vi "Main.vi"() -> ()   [LabVIEW 2013]
uses:
  <vilib>/myRIO/Instrument Drivers/Onboard IO/AI/vis/Smart Open.vi
  <vilib>/myRIO/Instrument Drivers/Onboard IO/AI/vis/Read.vi
  <vilib>/myRIO/Common/Instrument Driver Framework/myRIO v1.0/UART/vis/myRIO v1.0 Close UART.vi
  <vilib>/myRIO/Instrument Drivers/Onboard IO/AI/vis/Open.vi
  <vilib>/myRIO/Common/Instrument Driver Framework/myRIO v1.0/AI/vis/myRIO v1.1 Open AI.vi
  <vilib>/myRIO/Common/Instrument Driver Framework/Utilities/vis/Validate Channels.vi
  <vilib>/myRIO/Common/Instrument Driver Framework/myRIO v1.0/AI/vis/myRIO v1.0 Reserve AI.vi
  <vilib>/myRIO/Common/Instrument Driver Framework/myRIO v1.0/AI/vis/myRIO v1.0 Build MUX Configuration AI.vi
  <vilib>/myRIO/Common/Instrument Driver Framework/myRIO v1.0/Resource Manager/vis/myRIO v1.0 Reserve Channel List.vi
  <vilib>/myRIO/Common/Instrument Driver Framework/myRIO v1.0/Resource Manager/vis/myRIO v1.0 Reserve Channel.vi
  <vilib>/myRIO/Common/Instrument Driver Framework/myRIO v1.0/Resource Manager/vis/myRIO v1.0 Unreserve Channel.vi
  <vilib>/myRIO/Common/Instrument Driver Framework/myRIO v1.0/Resource Manager/vis/myRIO v1.0 Build Mutex Name.vi
  <vilib>/myRIO/Common/Instrument Driver Framework/myRIO v1.0/myRIO v1.1 Open.vi
  <vilib>/myRIO/Common/Instrument Driver Framework/myRIO v1.0/AI/vis/myRIO v1.0 Get Scaling Constants AI.vi
  <vilib>/Utility/VariantDataType/GetNumericInfo.vi
  <vilib>/Utility/error.llb/Error Cluster From Error Code.vi
  <vilib>/myRIO/Common/Instrument Driver Framework/Utilities/vis/IO Manager.vi
  <vilib>/myRIO/Common/Instrument Driver Framework/Utilities/vis/Configuration Manager.vi
  <vilib>/myRIO/Common/Instrument Driver Framework/myRIO v1.0/myRIO v1.0 Close.vi
  <vilib>/myRIO/Common/Instrument Driver Framework/myRIO v1.0/AI/vis/myRIO v1.0 Read AI.vi
  <vilib>/myRIO/Common/Instrument Driver Framework/Utilities/vis/FPGA Ref Manager.vi
  <vilib>/myRIO/Common/Instrument Driver Framework/myRIO v1.0/myRIO v1.0 Reset FPGA.vi
  <vilib>/myRIO/Instrument Drivers/Utilities/Utilities.lvlib
  <vilib>/ptbypt/NI_PtbyPt.lvlib
panel:
  out "numeric":dbl format="%_3g"
  in  "Koffset [cm]":dbl
  in  "Kscale [cm-V]":dbl=27.5
  out "Vo [V]":dbl format="%.2f"
  out "Range [cm]":dbl(knob) scale=0.0..80.0
  in  "[ESC]":bool
  # "IR Range Finder demo"
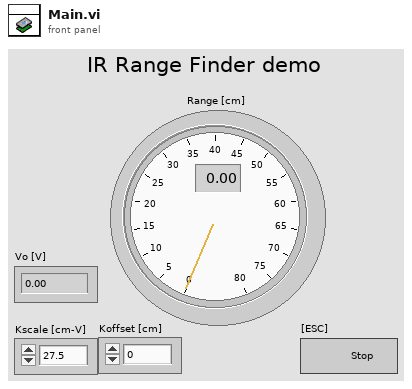
[diagram p1: front panel]
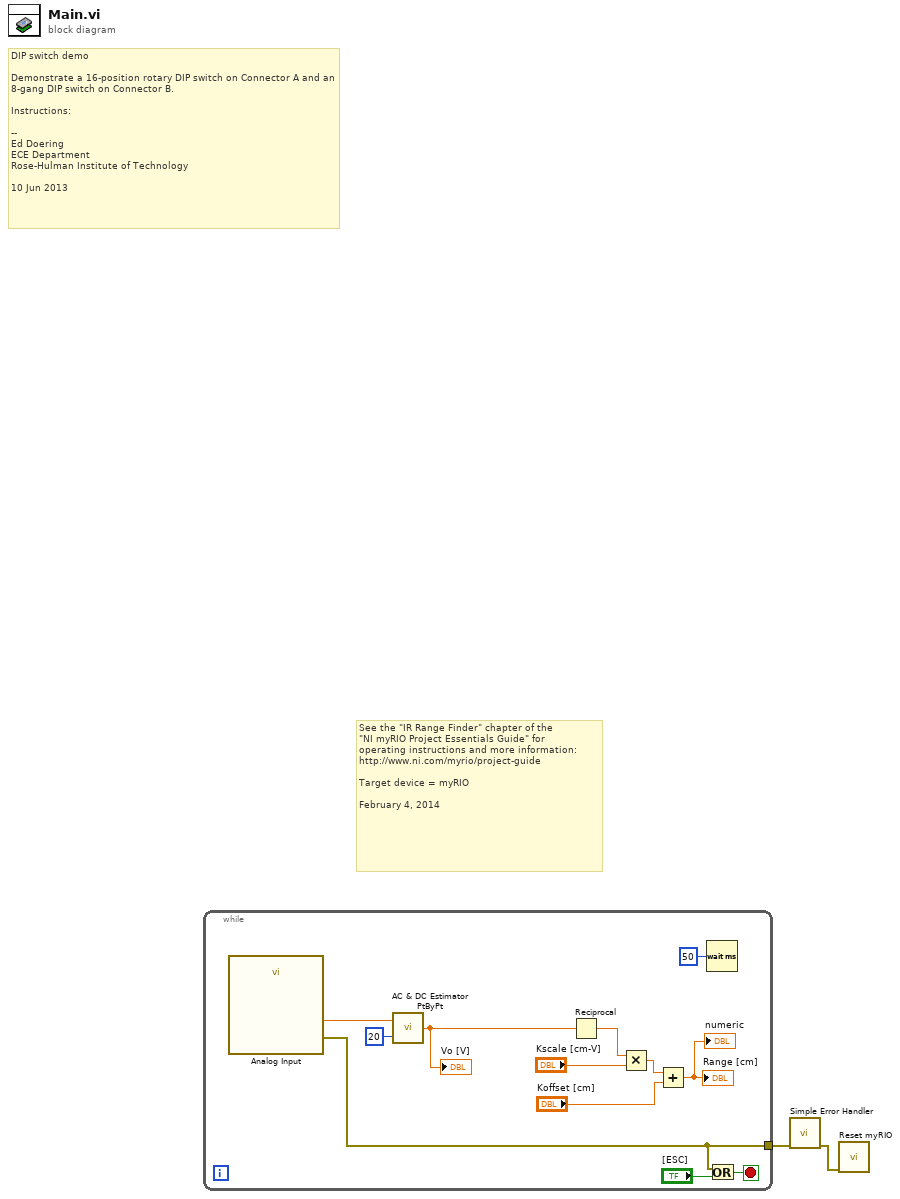
[diagram p0: block diagram]
diagram:
  # "See the \"IR Range Finder\" chapter of the\n\"NI myRIO Project Essentials Guide\" for\noperating instructions and more information: \nhttp://www.ni.com/myrio/project-guide\n\nTarget device = myRIO\n\nFebruary 4, 2014"
  # "DIP switch demo\n\nDemonstrate a 16-position rotary DIP switch on Connector A and an 8-gang DIP switch on Connector B.\n\nInstructions:\n\n-- \nEd Doering\nECE Department\nRose-Hulman Institute of Technology\n\n10 Jun 2013"
  n1 = while {
    tunnel: [w11] -> w1
    stop <- w13 stop-if-true
    n2 = call "Analog Input"() -> ("B/AI0 (Pin 3)"=w8:dbl, "error out"=w11:errorcluster)  [unwired: 26 in]
    n3 = call <vilib>:"AC & DC Estimator PtByPt.vi"("signal"=w8, "sample length"=20) -> ("DC estimate (V)"=w7:dbl)  [unwired: 1 in, 2 out]
    "Vo [V]" <- w7
    n4 = Reciprocal(x=w7) -> (1/x=w10:dbl)
    n5 = Multiply(x=w10, y="Kscale [cm-V]") -> (x*y=w4:dbl)
    n6 = Add(x=w4, y="Koffset [cm]") -> (x+y=→"Range [cm]" →"numeric":dbl)
    n7 = Wait (ms)(milliseconds to wait=u32 50) -> ()  [unwired: 1 out]
    n8 = Or(x=w11, y="[ESC]") -> (x .or. y?=w13:bool)
  }
  n9 = call <vilib>:"Simple Error Handler.vi"("error in (no error)"=w1) -> ("error out"=w2:errorcluster)  [unwired: 4 in, 4 out]
  n10 = call <vilib>:"Reset myRIO.vi"("error in (no error)"=w2) -> ()  [unwired: 10 in, 1 out]
